vi "auton_test.vi"(8 "FPGA VI Reference In":T1, 9 "reinit":bool, 10 "bus_inputs":T2, 11 "bus_state":T3) -> (2 "bus_inputs out":T2, 3 "bus_state out":T3)   [LabVIEW 2013]
uses:
  drivetrain/dt_shift_state.ctl
  <vilib>/Rock Robotics/SystemInterfaces/System/FPGA_SystemFRC FPGA Ref.ctl
  <vilib>/rvi/interface/nirviReadWriteControl/nirviReadWriteControl.xnode
  <vilib>/Rock Robotics/SystemInterfaces/FRC_FPGA_2012_1.6.4.lvbitx
  roller/roller_des_state.ctl
  NiFpgaLv.dll
  <vilib>/Utility/error.llb/Error Cluster From Error Code.vi
  <vilib>/rvi/errors/niLvFpgaAdjustHostInterfaceError.vi
  structures/bus_state_drivetrain.ctl
  structures/bus_state_collector.ctl
  structures/bus_state.ctl
  structures/bus_inputs.ctl
  collector/collector_shot_cal.ctl
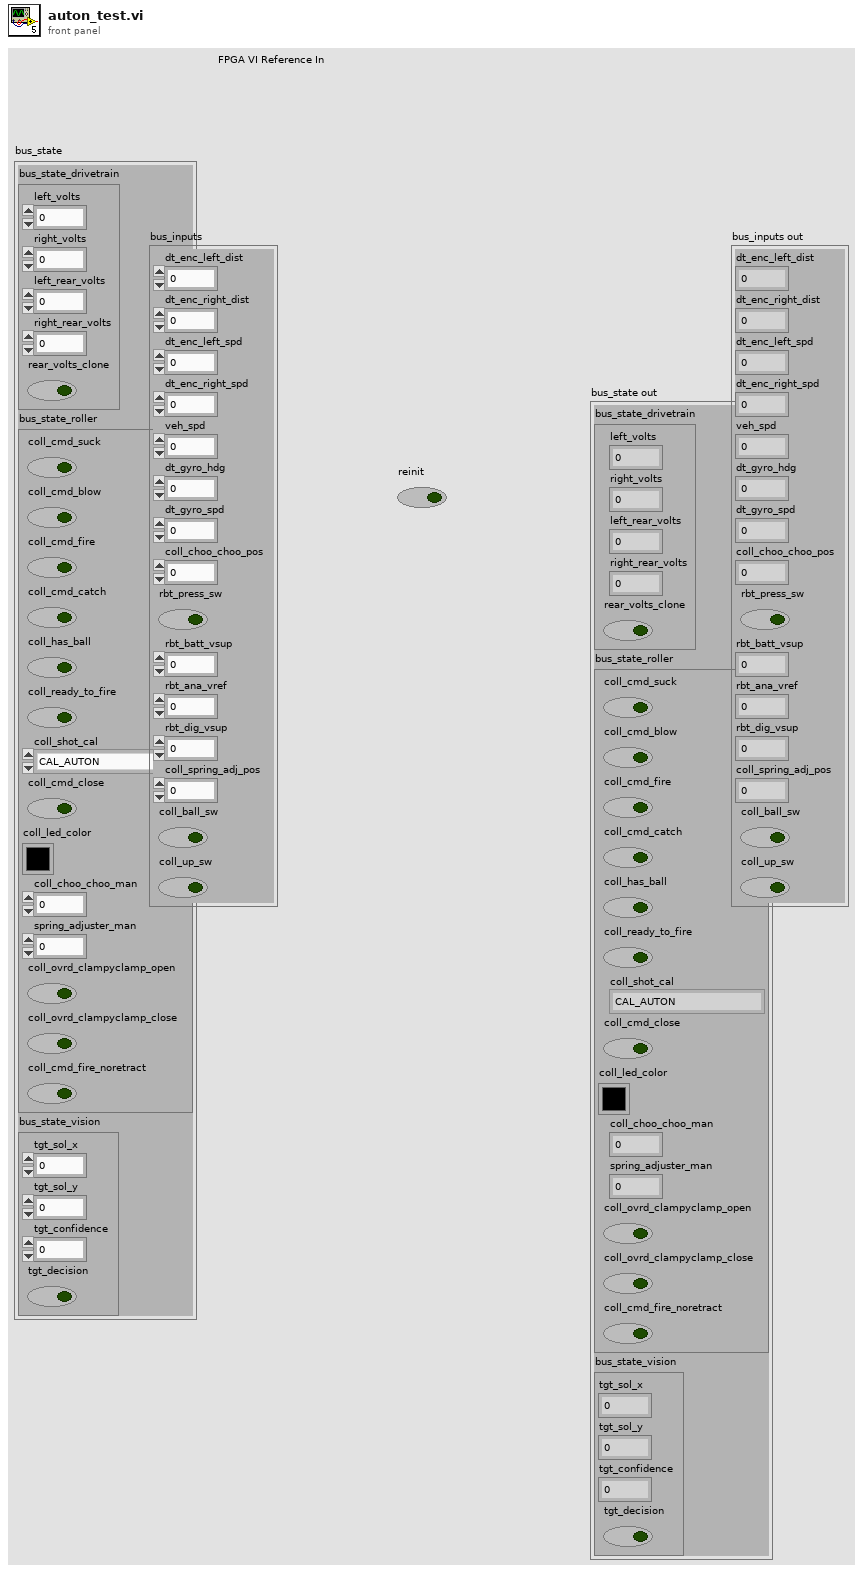
[diagram p1: front panel]
types:
  T1 = typedef "FPGA_SystemFRC FPGA Ref.ctl" = refnum<k20>
  T2 = typedef "bus_inputs.ctl" = cluster{"dt_enc_left_dist":sgl, "dt_enc_right_dist":sgl, "dt_enc_left_spd":sgl, "dt_enc_right_spd":sgl, "veh_spd":sgl, "dt_gyro_hdg":sgl, "dt_gyro_spd":sgl, "coll_choo_choo_pos":sgl, "rbt_press_sw":bool, "rbt_batt_vsup":sgl, "rbt_ana_vref":dbl, "rbt_dig_vsup":dbl, "coll_spring_adj_pos":sgl, "coll_ball_sw":bool, "coll_up_sw":bool}
  T3 = typedef "bus_state.ctl" = cluster{"bus_state_drivetrain":T4, "bus_state_roller":T5, "bus_state_vision":cluster{"tgt_sol_x":dbl, "tgt_sol_y":dbl, "tgt_confidence":dbl, "tgt_decision":bool}}
  T4 = typedef "bus_state_drivetrain.ctl" = cluster{"left_volts":sgl, "right_volts":sgl, "left_rear_volts":sgl, "right_rear_volts":sgl, "rear_volts_clone":bool}
  T5 = typedef "bus_state_collector.ctl" = cluster{"coll_cmd_suck":bool, "coll_cmd_blow":bool, "coll_cmd_fire":bool, "coll_cmd_catch":bool, "coll_has_ball":bool, "coll_ready_to_fire":bool, "coll_shot_cal":T6, "coll_cmd_close":bool, "coll_led_color":u32, "coll_choo_choo_man":sgl, "spring_adjuster_man":sgl, "coll_ovrd_clampyclamp_open":bool, "coll_ovrd_clampyclamp_close":bool, "coll_cmd_fire_noretract":bool}
  T6 = typedef "collector_shot_cal.ctl" = enum16{"CAL_AUTON", "CAL_CLOSE", "CAL_MID", "CAL_FAR", "NOT_SAFE_TO_ACTUATE"}
  T7 = typedef "roller_des_state.ctl" = enum16{"OFF", "SUCK", "BLOW"}
  T8 = typedef "dt_shift_state.ctl" = enum16{"low", "high"}
  T9 = cluster{"dt_enc_right_dist":sgl, "dt_enc_right_dist":sgl}
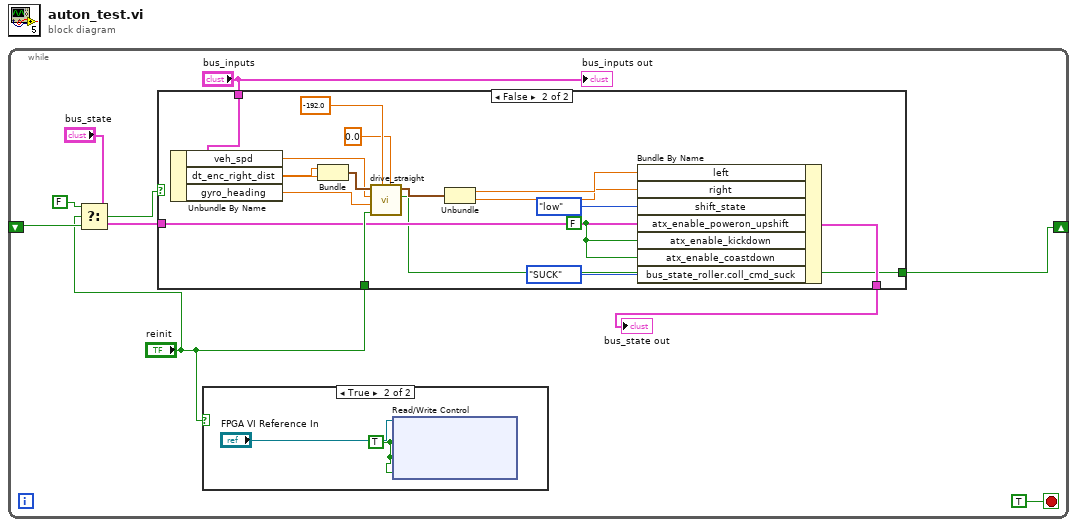
[diagram p0: block diagram]
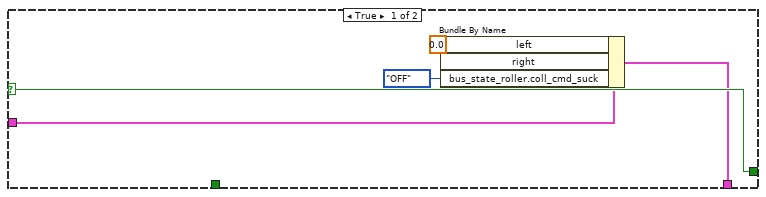
[diagram p3: hidden frame]
diagram:
  n1 = while {
    shift-right: [w2] -> _
    shift-left: _ -> [w5]
    stop <- TRUE stop-if-true
    n2 = Select(t=FALSE, s="reinit", f=w5) -> (s? t:f=w4:bool)
    n3 = case shown="False" w4 {
      selector: w4 -> [w16 _]
      tunnel: "reinit" -> [_ w30]
      tunnel: "bus_state" -> [w15 w26]
      tunnel: "bus_inputs" -> [_ w25]
      tunnel: [w14 w21] -> w7
      tunnel: [w16 w18] -> w2
      frame True {
        w13 = 0.0 ("bus_state_drivetrain.left")
        n4 = Bundle By Name(cluster=w15, "left"=w13, "right"=w13, "bus_state_roller.coll_cmd_suck"=roller_des_state."OFF" ("bus_state_roller.roller_des_state")) -> (w14:T3)
      }
      frame False {
        w20 = FALSE ("bus_state_drivetrain.atx_enable_poweron_upshift")
        n5 = Unbundle By Name(w25) -> ("veh_spd"=w31:sgl, "dt_enc_right_dist"=w33:sgl, "gyro_heading"=w29:dbl)
        n6 = Bundle("dt_enc_right_dist"=w33, "dt_enc_right_dist"=w33) -> (w32:T9)  [unwired: 1 in]
        n7 = call "drive_straight.vi"("setpoint_hdg"=0.0, "setpoint_distance"=-192.0, "reinit"=w30, "gyro_heading"=w29, "vehspd_avg"=w31, "distances"=w32) -> ("done"=w18:bool, "mpower"=w24:cluster{"left":dbl, "right":dbl})  [unwired: 4 in]
        n8 = Unbundle(w24) -> ("left"=w23:dbl, "right"=w22:dbl)
        n9 = Bundle By Name(cluster=w26, "left"=w23, "right"=w22, "shift_state"=dt_shift_state."low" ("bus_state_drivetrain.shift_state"), "atx_enable_poweron_upshift"=w20, "atx_enable_kickdown"=w20, "atx_enable_coastdown"=w20, "bus_state_roller.coll_cmd_suck"=roller_des_state."SUCK" ("bus_state_roller.roller_des_state")) -> (w21:T3)
      }
    }
    "bus_state out" <- w7
    n10 = case shown="True" "reinit" {
      frame False {
      }
      frame True {
        w10 = TRUE ("Encoder0.Reset")
        n11 = xnode "Read/Write Control"("FPGA VI Reference In"="FPGA VI Reference In", "Encoder0.Reset"=w10, "Encoder1.Reset"=w10, "Accumulator0.Reset"=w10) -> ()  [unwired: 1 in, 2 out]
      }
    }
    "bus_inputs out" <- "bus_inputs"
  }
